vi "Host - Thruster signal (SubVI).vi"(10 "T Status":bool) -> (2 "T - Signal":bool)   [LabVIEW 2021]
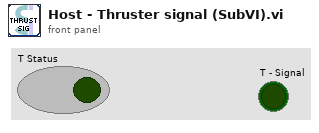
[diagram p1: front panel]
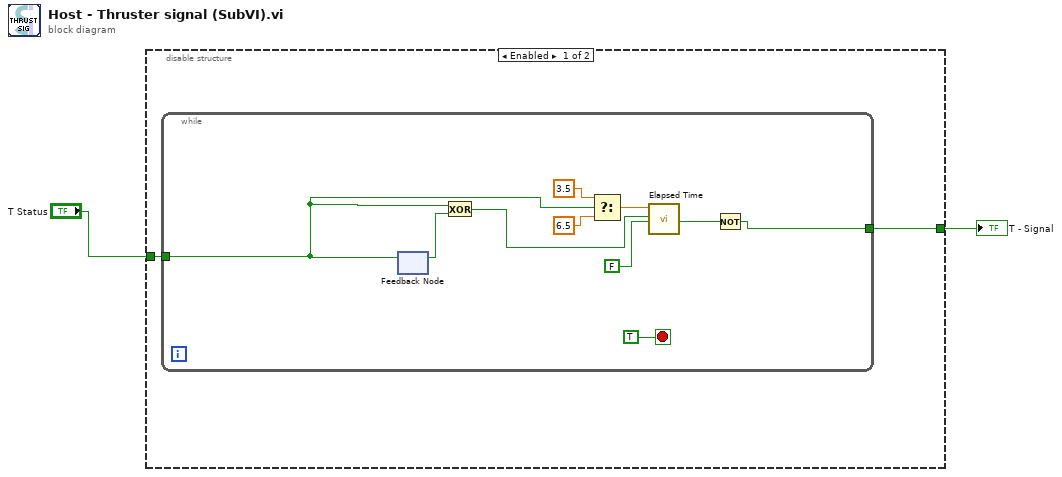
[diagram p0: block diagram]
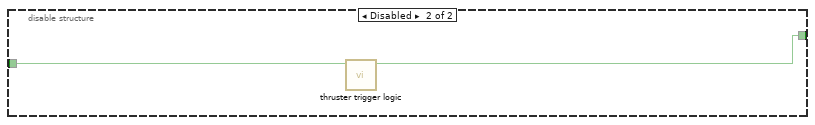
[diagram p2: hidden frame]
diagram:
  n1 = disable-structure shown="Enabled" {
    disable-tunnel: "T Status" -> [w4 w16]
    disable-tunnel: [w3 w15] -> w1
    frame Enabled {
      n2 = while {
        tunnel: w4 -> [w6]
        tunnel: [w5] -> w3
        stop <- TRUE stop-if-true
        n3 = feedback-in #1(w6) -> ()
        n4 = feedback #1() -> (w10:bool)  [unwired: 1 in]
        n5 = Exclusive Or(1:w10, 2:w6) -> (0:w9:bool)
        n6 = Select(t=3.5 ("y"), s=w6, f=6.5 ("y")) -> (s? t:f=w12:dbl)
        n7 = call "Elapsed Time"("Time Target (s)"=w12, "Reset"=w9, "Auto Reset"=FALSE) -> ("Time has Elapsed"=w13:bool)  [unwired: 9 in, 7 out]
        n8 = Not(x=w13) -> (.not. x?=w5:bool)
      }
    }
    frame Disabled {
      n9 = call "thruster trigger logic.vi"("control"=w16) -> ("signal"=w15:bool)  [unwired: 9 in, 1 out]
    }
  }
  "T - Signal" <- w1
